vi "Slider Position Chasing Top Max.vi"(5 "Asigned Slider":i32=1, 7 "Chasing Active Slider":bool=TRUE, 8 "Position Compensate":cluster{"Array 2":dbl[]}[](array[cluster]) {"Array 2" format="%#_f"}, 10 "Chasing Group":cluster{"Array 2":refnum<vi>[]}[](array[cluster]), 11 "Slide Reference In":refnum<vi>) -> (3 "Slide Reference Out":refnum<vi>)   [LabVIEW 2024]
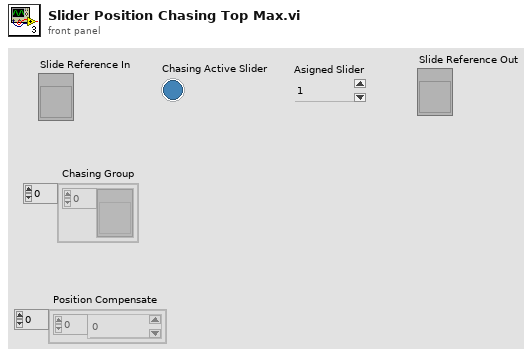
[diagram p1: front panel]
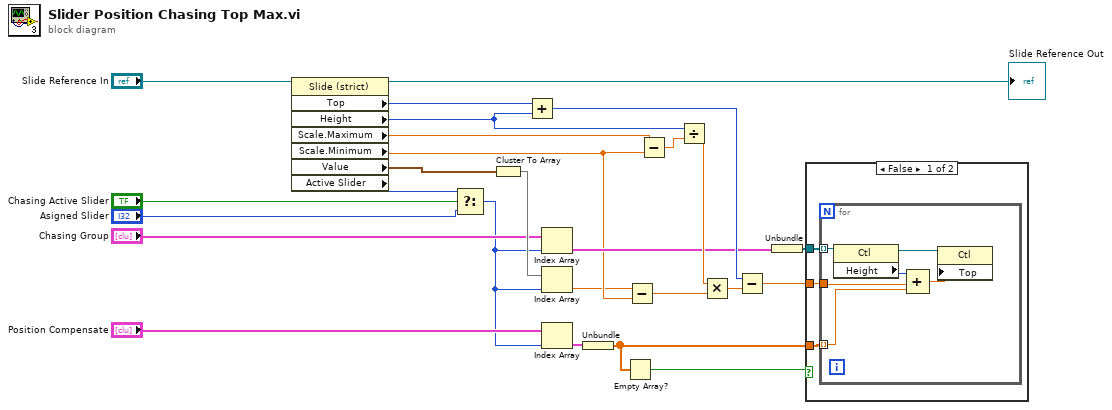
[diagram p0: block diagram]
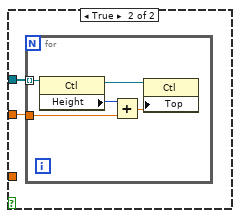
[diagram p2: hidden frame]
diagram:
  n1 = property class="Slide (strict)"(reference="Slide Reference In") -> (reference out=→"Slide Reference Out":refnum<vi>, "Top"=w25:i32, "Height"=w24:u32, "Scale.Maximum"=w4:dbl, "Scale.Minimum"=w2:dbl, "Value"=w18:cluster{dbl, dbl, dbl}, "Active Slider"=w7:i32)  [unwired: 1 in, 1 out]
  n2 = Select(t=w7, s="Chasing Active Slider", f="Asigned Slider") -> (s? t:f=w6:i32)
  n3 = Cluster To Array(cluster=w18) -> (array=w17:dbl[])
  n4 = Add(x=w25, y=w24) -> (x+y=w21:u32)
  n5 = Index Array(array="Chasing Group", index=w6) -> (element=w15:cluster{"Array 2":refnum<vi>[]})
  n6 = Index Array(array=w17, index=w6) -> (element=w1:dbl)
  n7 = Index Array(array="Position Compensate", index=w6) -> (element=w12:cluster{"Array 2":dbl[]})
  n8 = Unbundle(w12) -> ("Array 2"=w10:dbl[])
  n9 = Empty Array?(array=w10) -> (empty?=w11:bool)
  n10 = Subtract(x=w1, y=w2) -> (x-y=w3:dbl)
  n11 = Subtract(x=w4, y=w2) -> (x-y=w26:dbl)
  n12 = Divide(x=w24, y=w26) -> (x/y=w22:dbl)
  n13 = Multiply(x=w22, y=w3) -> (x*y=w23:dbl)
  n14 = Subtract(x=w21, y=w23) -> (x-y=w20:dbl)
  n15 = Unbundle(w15) -> ("Array 2"=w14:refnum<vi>[])
  n16 = case shown="False" w11 {
    tunnel: w20 -> [w29 w36]
    tunnel: w14 -> [w28 w37]
    tunnel: w10 -> [w27 _]
    frame False {
      n17 = for {
        tunnel: w29 -> [w31]
        tunnel: w28 -> [w32] mode=indexing
        tunnel: w27 -> [w30] mode=indexing
        n18 = property class="Ctl"(reference=w32) -> (reference out=w34:refnum<vi>, "Height"=w33:u32)  [unwired: 1 in, 1 out]
        n19 = Compound Arithmetic op=ADD(w33, w31, w30) -> (w35:dbl)
        n20 = property class="Ctl"(reference=w34, "Top"=w35) -> ()  [unwired: 1 in, 2 out]
      }
    }
    frame True {
      n21 = for {
        tunnel: w36 -> [w40]
        tunnel: w37 -> [w41] mode=indexing
        n22 = property class="Ctl"(reference=w41) -> (reference out=w42:refnum<vi>, "Height"=w39:u32)  [unwired: 1 in, 1 out]
        n23 = Add(x=w39, y=w40) -> (x+y=w38:dbl)
        n24 = property class="Ctl"(reference=w42, "Top"=w38) -> ()  [unwired: 1 in, 2 out]
      }
    }
  }
